vi "Two LightField Instances.vi"() -> ()   [LabVIEW 2015]
uses:
  lightfield-automation-labview/LightField Automation.lvclass
panel:
  in  "ExperimentName 2":string
  in  "ExperimentName":string
  in  "stop":bool
  in  "Exposure Time (s) 2":dbl(knob)=92.509 step=0.001 scale=0.0..1000.0
  in  "Exposure Time (s)":dbl(knob)=430.129 step=0.001 scale=0.0..1000.0
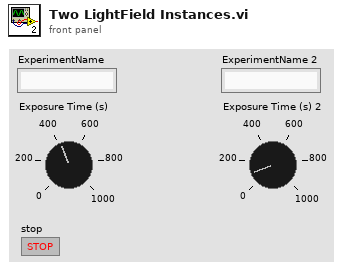
[diagram p1: front panel]
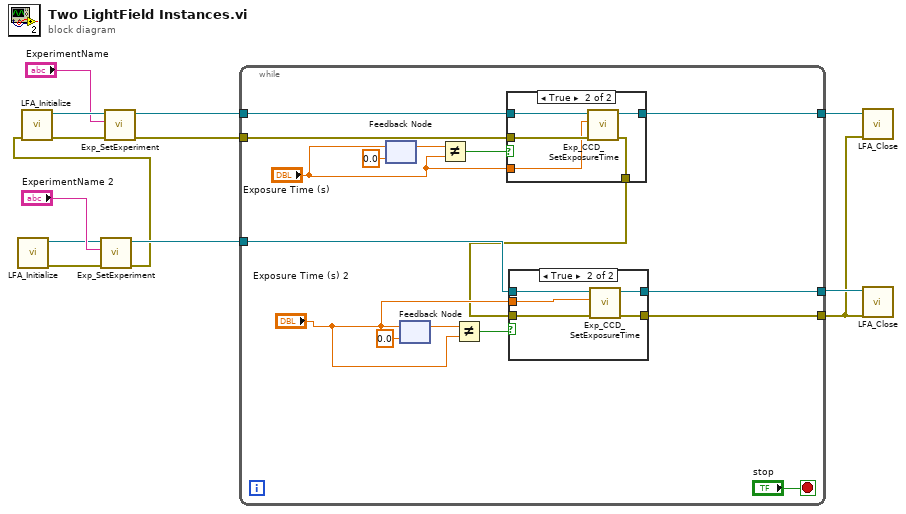
[diagram p0: block diagram]
diagram:
  n1 = call "LFA_Initialize.vi"() -> ("error out"=w8:errorcluster, "LightField Automation out"=w7:refnum<class "LightField Automation.lvclass">)  [unwired: 10 in]
  n2 = call "Exp_SetExperiment.vi"("error in (no error)"=w8, "ExperimentName"="ExperimentName 2", "LightField Automation in"=w7) -> ("error out"=w5:errorcluster, "LightField Automation out"=w6:refnum<class "LightField Automation.lvclass">)  [unwired: 7 in]
  n3 = call "LFA_Initialize.vi"("error in (no error)"=w5) -> ("error out"=w12:errorcluster, "LightField Automation out"=w13:refnum<class "LightField Automation.lvclass">)  [unwired: 9 in]
  n4 = call "Exp_SetExperiment.vi"("error in (no error)"=w12, "ExperimentName"="ExperimentName", "LightField Automation in"=w13) -> ("error out"=w4:errorcluster, "LightField Automation out"=w10:refnum<class "LightField Automation.lvclass">)  [unwired: 7 in]
  n5 = while {
    tunnel: w6 -> [w20]
    tunnel: w10 -> [w26]
    tunnel: w4 -> [w25]
    tunnel: [w18] -> w2
    tunnel: [w17] -> w3
    tunnel: [w16] -> w1
    stop <- "stop" stop-if-true
    n6 = feedback-in #1("Exposure Time (s)") -> ()
    n7 = feedback #1(0.0 ("Exposure Time (s)")) -> (w29:dbl)
    n8 = feedback #2(0.0 ("Exposure Time (s)")) -> (w23:dbl)
    n9 = feedback-in #2("Exposure Time (s) 2") -> ()
    n10 = Not Equal?(x=w29, y="Exposure Time (s)") -> (x != y?=w27:bool)
    n11 = Not Equal?(x=w23, y="Exposure Time (s) 2") -> (x != y?=w22:bool)
    n12 = case shown="True" w27 {
      tunnel: w26 -> [w37 w43]
      tunnel: w25 -> [w38 w42]
      tunnel: [w38 w41] -> w19
      tunnel: [w37 w40] -> w18
      tunnel: "Exposure Time (s)" -> [_ w39]
      frame False {
      }
      frame True {
        n13 = call "Exp_CCD_SetExposureTime.vi"("error in (no error)"=w42, "Exposure Time (s)"=w39, "LightField Automation in"=w43) -> ("error out"=w41:errorcluster, "LightField Automation out"=w40:refnum<class "LightField Automation.lvclass">)  [unwired: 7 in]
      }
    }
    n14 = case shown="True" w22 {
      tunnel: w20 -> [w31 w36]
      tunnel: w19 -> [w30 w35]
      tunnel: "Exposure Time (s) 2" -> [_ w34]
      tunnel: [w31 w33] -> w17
      tunnel: [w30 w32] -> w16
      frame False {
      }
      frame True {
        n15 = call "Exp_CCD_SetExposureTime.vi"("error in (no error)"=w35, "Exposure Time (s)"=w34, "LightField Automation in"=w36) -> ("error out"=w32:errorcluster, "LightField Automation out"=w33:refnum<class "LightField Automation.lvclass">)  [unwired: 7 in]
      }
    }
  }
  n16 = call "LFA_Close.vi"("error in (no error)"=w1, "LightField Automation in"=w2) -> ()  [unwired: 8 in, 2 out]
  n17 = call "LFA_Close.vi"("error in (no error)"=w1, "LightField Automation in"=w3) -> ()  [unwired: 8 in, 2 out]
